vi "PSK_change_code.vi"(8 "error in (no error)":errorcluster caption="错误输入（无错误）", 10 "input_data":dbl[](array[numeric]) format="%#_13g", 11 "PathIn":path) -> (0 "error out":errorcluster caption="错误输出", 3 "PathOut":path, 6 "x":dbl[](array[numeric]))   [LabVIEW 2015]
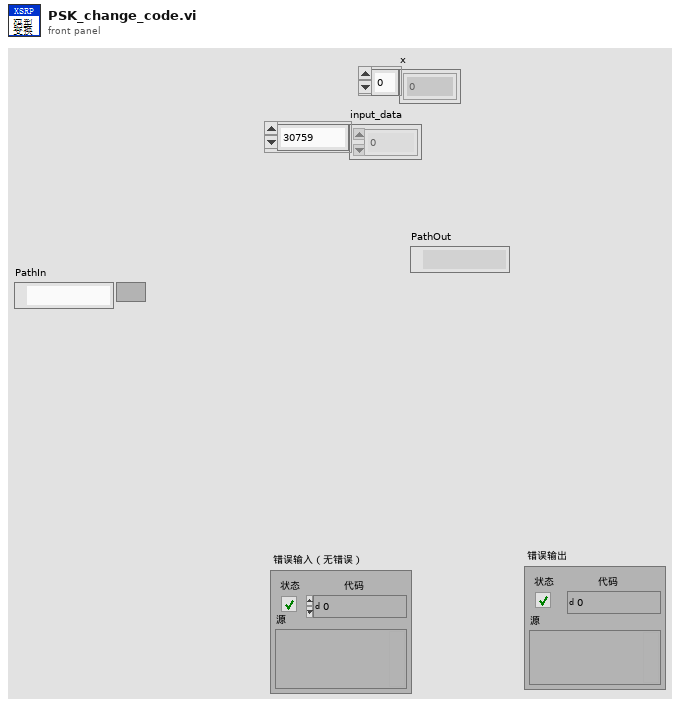
[diagram p1: front panel]
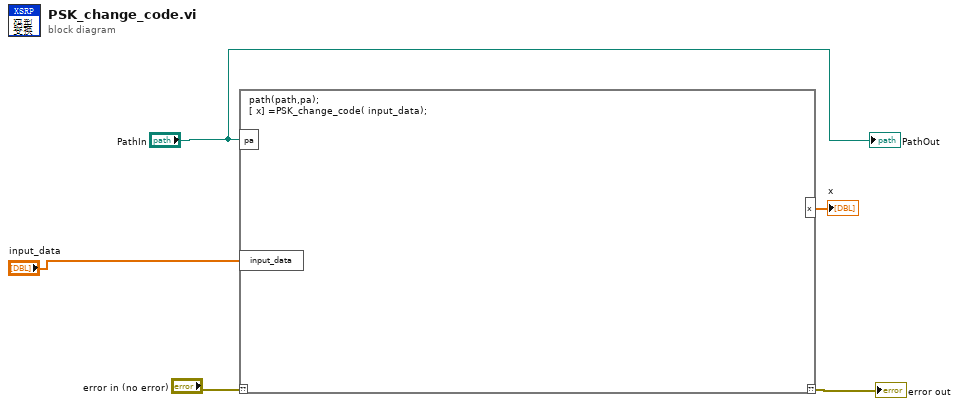
[diagram p0: block diagram]
diagram:
  n1 = script code="path(path,pa);\n[ x] =PSK_change_code( input_data);"("??"="error in (no error)", "pa"="PathIn", "input_data"="input_data") -> ("??"=→"error out":errorcluster, "x"=→"x":dbl[])
  "PathOut" <- "PathIn"
